vi "interv2.vi"(0 "pixel x1":i32, 1 "Pixel x2":i32, 2 "pixel y1":i32, 3 "pixel y2":i32, 4 "esp. x1":dbl, 5 "esp. x2":dbl, 6 "esp. y1":dbl, 7 "esp. y2":dbl) -> (21 "paso x":dbl, 24 "paso y":dbl)   [LabVIEW 2016]
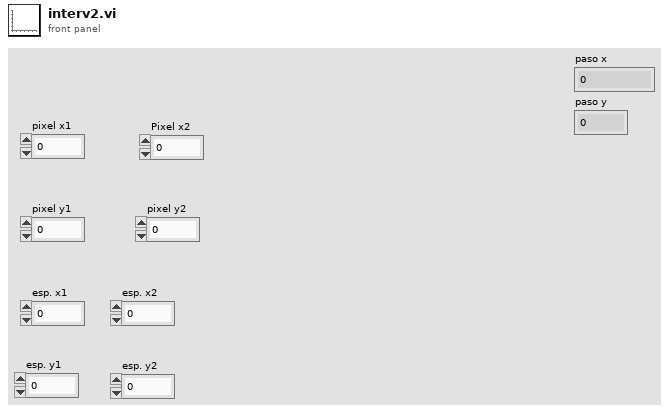
[diagram p1: front panel]
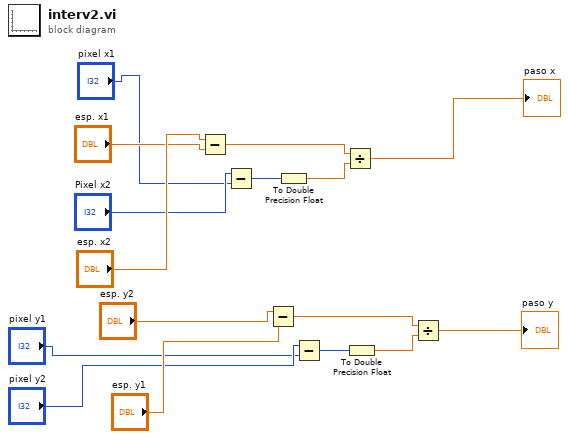
[diagram p0: block diagram]
diagram:
  n1 = Subtract(x="esp. x2", y="esp. x1") -> (x-y=w12:dbl)
  n2 = Subtract(x="Pixel x2", y="pixel x1") -> (x-y=w11:i32)
  n3 = Subtract(x="esp. y2", y="esp. y1") -> (x-y=w8:dbl)
  n4 = To Double Precision Float(number=w11) -> (double precision float=w10:dbl)
  n5 = Subtract(x="pixel y2", y="pixel y1") -> (x-y=w7:i32)
  n6 = Divide(x=w12, y=w10) -> (x/y=→"paso x":dbl)
  n7 = To Double Precision Float(number=w7) -> (double precision float=w6:dbl)
  n8 = Divide(x=w8, y=w6) -> (x/y=→"paso y":dbl)
